vi "listener mode.vi"() -> ()   [LabVIEW 2014]
uses:
  <vilib>/userdefined/High Color/IMAQdx.ctl
  <vilib>/vision/driver/IMAQdx.llb/IMAQdx Camera Control Mode.ctl
  <vilib>/vision/driver/NI_Vision_Acquisition_Software.lvlib
panel:
  out "error out 2":errorcluster
  out "error out":errorcluster
  in  "Boolean":bool
  out "Image":T1(plugin-control)
  in  "IMAQdx Session":T2
  # "Bei der Camera muss\nals Broadcast oder \nMulticast eingestellt\nsein!"
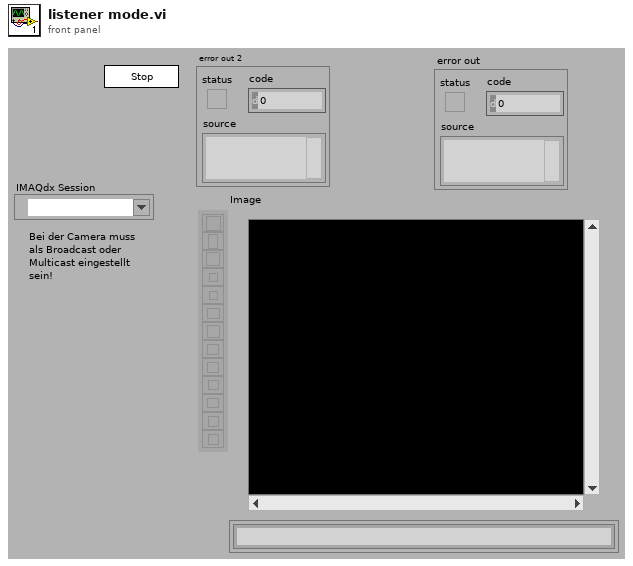
[diagram p1: front panel]
types:
  T1 = typedef "IMAQ Image.ctl" = refnum<image>
  T2 = typedef "IMAQdx.ctl" = refnum<k21>
  T3 = typedef "NI_Vision_Acquisition_Software.lvlib/IMAQdx Camera Control Mode.ctl" = enum32{"Controller", "Listener"}
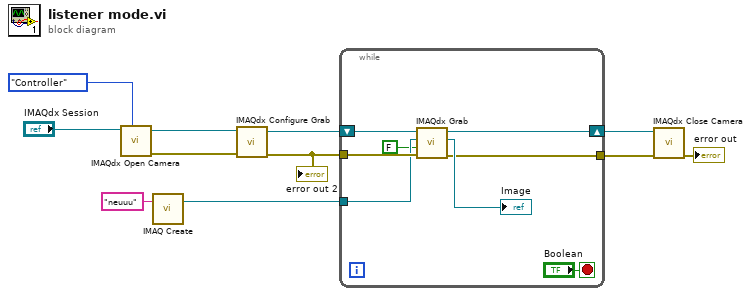
[diagram p0: block diagram]
diagram:
  n1 = call <vilib>:"IMAQdx Open Camera.vi"("Camera Control Mode"=IMAQdx_Camera_Control_Mode."Controller", "Session In"="IMAQdx Session") -> ("error out"=w8:errorcluster, "Session Out"=w9:T2)  [unwired: 8 in]
  n2 = call "IMAQ Create"("Image Name"="neuuu") -> ("New Image"=w4:T1)  [unwired: 4 in, 1 out]
  n3 = call <vilib>:"IMAQdx Configure Grab.vi"("error in"=w8, "Session In"=w9) -> ("error out"=w6:errorcluster, "Session Out"=w7:T2)  [unwired: 8 in]
  "error out 2" <- w6
  n4 = while {
    tunnel: w6 -> [w18]
    tunnel: w4 -> [w17]
    shift-right: [w13] -> w2
    shift-left: w7 -> [w19]
    tunnel: [w14] -> w3
    stop <- "Boolean" stop-if-true
    n5 = call <vilib>:"IMAQdx Grab.vi"("error in"=w18, "Wait for Next Buffer? (Yes)"=FALSE, "Image In"=w17, "Session In"=w19) -> ("error out"=w14:errorcluster, "Image Out"=→"Image":T1, "Session Out"=w13:T2)  [unwired: 4 in, 1 out]
  }
  n6 = call <vilib>:"IMAQdx Close Camera.vi"("error in"=w3, "Session In"=w2) -> ("error out"=→"error out":errorcluster)  [unwired: 9 in]
